vi "LinkItemFromXML.vi"(11 "XML for one item":string) -> (3 "GettingStartedWindow.lvlib:Link.lvclass":refnum<class "Link.lvclass">)   [LabVIEW 2009, in "NavScreen.lvlib" / "Link.lvclass"]
uses:
  Link.lvclass
  Error/Error.lvclass
  NavScreen.lvlib
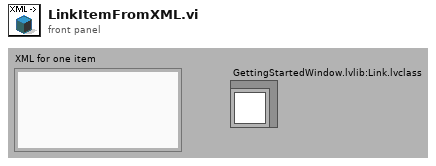
[diagram p1: front panel]
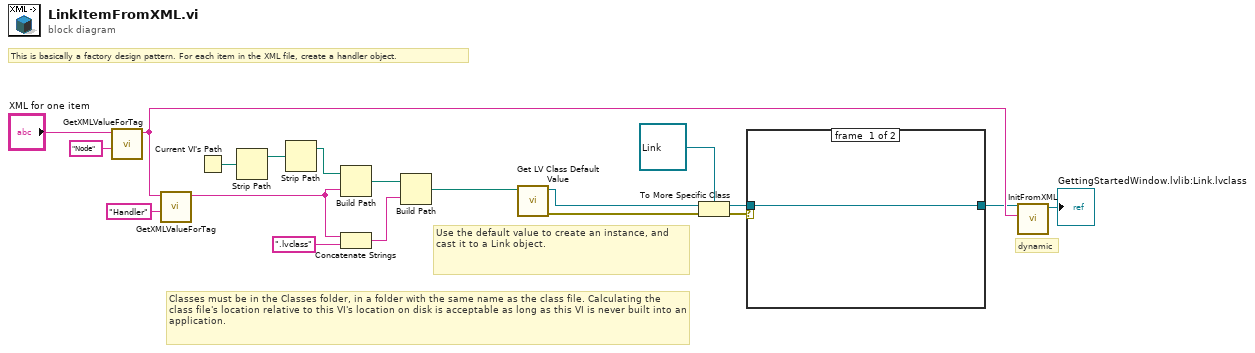
[diagram p0: block diagram]
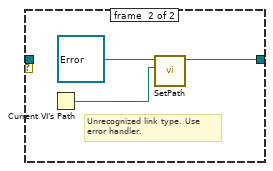
[diagram p2: hidden frame]
diagram:
  # "Use the default value to create an instance, and cast it to a Link object."
  # "Classes must be in the Classes folder, in a folder with the same name as the class file. Calculating the class file's location relative to this VI's location on disk is acceptable as long as this VI is never built into an application."
  # "This is basically a factory design pattern. For each item in the XML file, create a handler object."
  # "dynamic"
  n1 = call "GetXMLValueForTag.vi"("tag"="Node", "XML"="XML for one item") -> ("value"=w15:string)  [unwired: 8 in, 1 out]
  n2 = call "GetXMLValueForTag.vi"("tag"="Handler", "XML"=w15) -> ("value"=w11:string)  [unwired: 8 in, 1 out]
  n3 = Current VI's Path() -> (path=w14:path)
  n4 = Strip Path(path=w14) -> (stripped path=w13:path)  [unwired: 1 out]
  n5 = Strip Path(path=w13) -> (stripped path=w12:path)  [unwired: 1 out]
  n6 = Build Path(base path=w12, name or relative path=w11) -> (appended path=w9:path)
  n7 = Concatenate Strings(w11, ".lvclass" ("string")) -> (w8:string)
  n8 = Build Path(base path=w9, name or relative path=w8) -> (appended path=w3:path)
  n9 = call <vilib>:"Get LV Class Default Value.vi"("class path"=w3) -> ("error out"=w1:errorcluster, "object"=w2:refnum<class>)  [unwired: 9 in]
  n10 = To More Specific Class(target class=refnum<class "Link.lvclass"> refnum ("GettingStartedWindow.lvlib:Link.lvclass"), reference=w2, error in=w1) -> (specific class reference=w5:refnum<class "Link.lvclass">, error out=w6:errorcluster)
  n11 = case shown="No Error" w6 {
    tunnel: w5 -> [w20 _]
    tunnel: [w20 w21] -> w4
    frame #0 {
    }
    frame #1 {
      # "Unrecognized link type. Use\nerror handler."
      n12 = Current VI's Path() -> (path=w23:path)
      n13 = call "SetPath.vi"("path to VI that identifies classes"=w23, "GettingStartedWindow.lvlib:Error.lvclass"=refnum<class "Error.lvclass"> refnum) -> ("GettingStartedWindow.lvlib:Error.lvclass 2"=w21:refnum<class "Error.lvclass">)  [unwired: 9 in]
    }
  }
  n14 = call-dynamic "InitFromXML.vi"("XML"=w15, "Link in"=w4) -> ("Link out"=→"GettingStartedWindow.lvlib:Link.lvclass":refnum<class "Link.lvclass">)  [unwired: 8 in, 1 out]
